vi "Mathcad 15 writeV.vi"(8 "error in (no error)":errorcluster, 10 "file text":string, 11 "DesignRequest":T1={"Project Folder"=path "", "Method Name"="", "Inputs"=[{"Label.Text"="L.Box", "Control Type"=0, "Numeric"=5.0, "Array"=[], "status"=FALSE, "Str Array"=[], "String"="", "unit"="m"}, {"Label.Text"="W.Box", "Control Type"=0, "Numeric"=2.0, "Array"=[], "status"=FALSE, "Str Array"=[], "String"="", "unit"="m"}, {"Label.Text"="H.Box", "Control Type"=0, "Numeric"=11.0, "Array"=[], "status"=FALSE, "Str Array"=[], "String"="", "unit"="m"}], "Version"=0}) -> (0 "error out":errorcluster, 2 "file text out":string)   [LabVIEW 2012, in "Design Server.lvlib"]
uses:
  Design Server.lvlib
  Design Request.ctl
  Variable cluster.ctl
panel:
  out "unit":string
  out "Array":string[](array[string])
  out "indexes":i32[](array[numeric])
  out "Regions":string[](array[string])
  # "replace existing region"
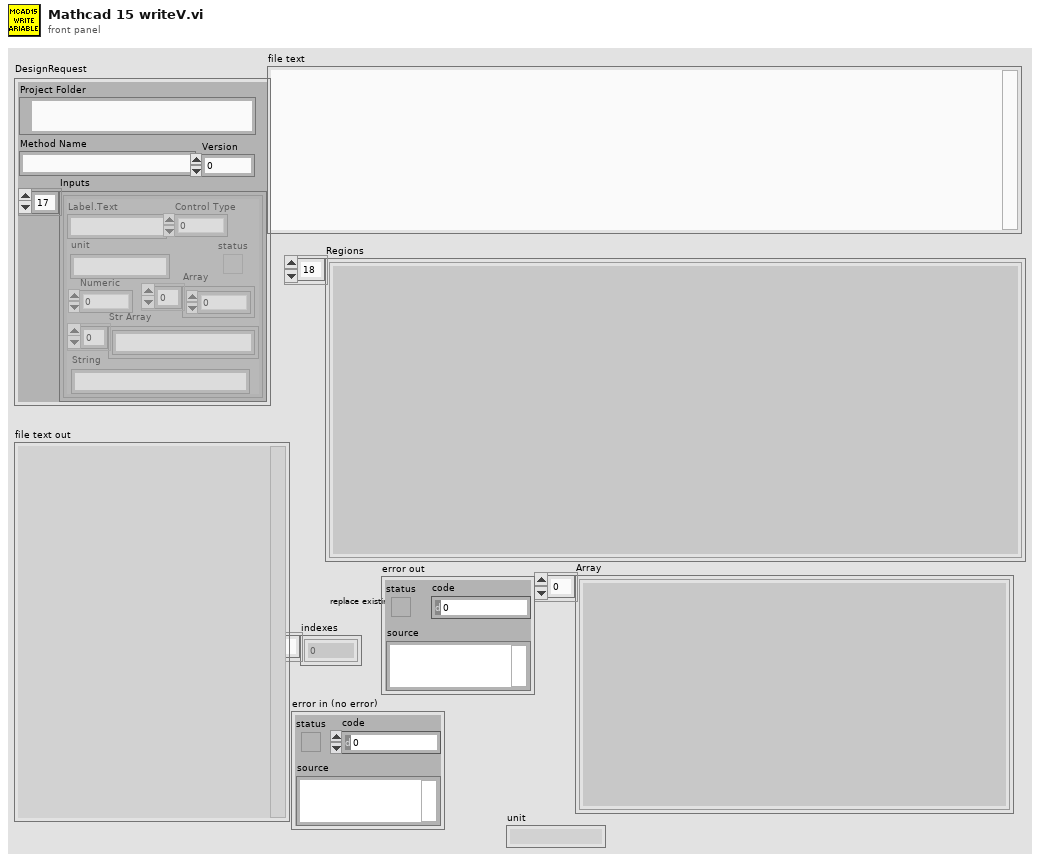
[diagram p1: front panel]
types:
  T1 = typedef "Design Server.lvlib/Design Request.ctl" = cluster{"Project Folder":path, "Method Name":string, "Inputs":T2, "Version":i32}
  T2 = typedef "Design Server.lvlib/Variable cluster.ctl" = cluster{"Label.Text":string, "Control Type":u32, "Numeric":dbl, "Array":dbl[], "status":bool, "Str Array":string[], "String":string, "unit":string}[]
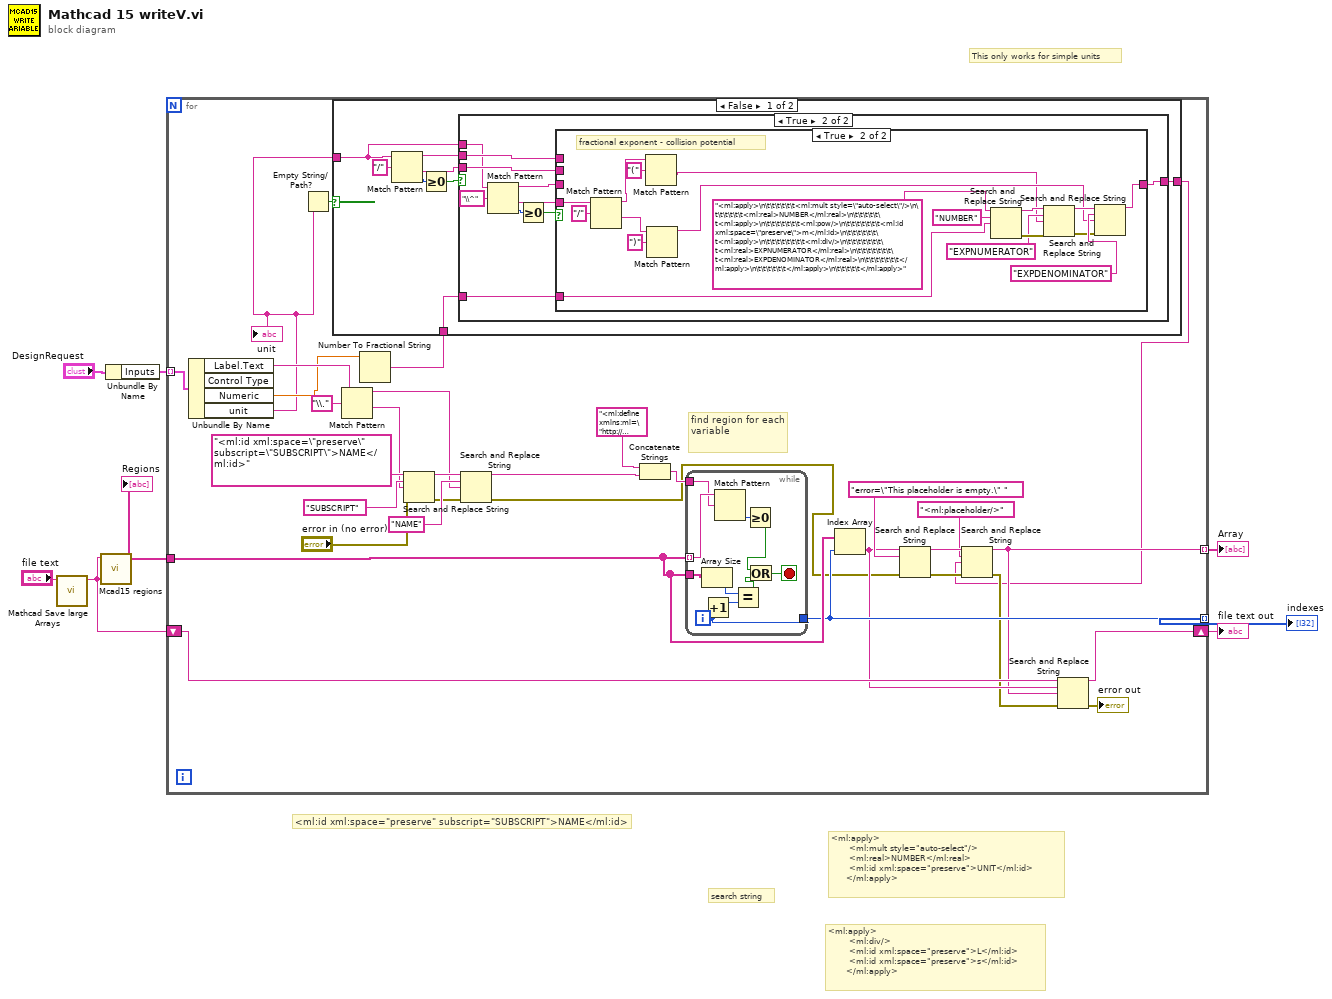
[diagram p0: block diagram]
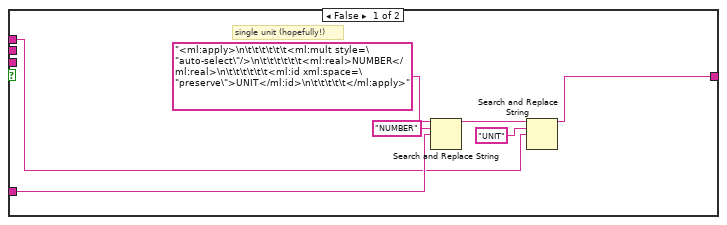
[diagram p2: hidden frame]
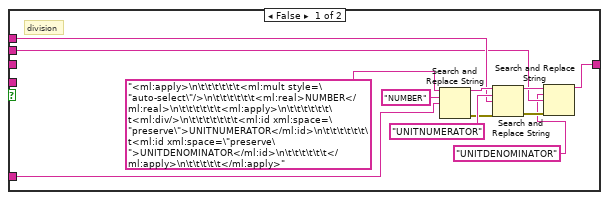
[diagram p3: hidden frame]
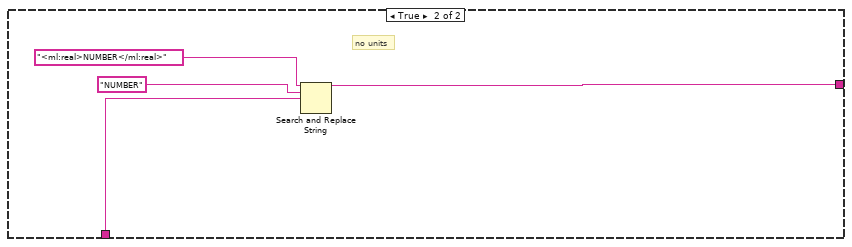
[diagram p4: hidden frame]
diagram:
  # "This only works for simple units"
  # "<ml:apply>\n\t\t\t\t\t\t\t<ml:div/>\n\t\t\t\t\t\t\t<ml:id xml:space=\"preserve\">L</ml:id>\n\t\t\t\t\t\t\t<ml:id xml:space=\"preserve\">s</ml:id>\n\t\t\t\t\t\t</ml:apply>"
  # "<ml:apply>\n\t\t\t\t\t\t<ml:mult style=\"auto-select\"/>\n\t\t\t\t\t\t<ml:real>NUMBER</ml:real>\n\t\t\t\t\t\t<ml:id xml:space=\"preserve\">UNIT</ml:id>\n\t\t\t\t\t</ml:apply>"
  # "search string"
  # "<ml:id xml:space=\"preserve\" subscript=\"SUBSCRIPT\">NAME</ml:id>"
  n1 = call "Mathcad Save large Arrays.vi"("file text"="file text") -> ("file text w save large arrays"=w1:string)  [unwired: 9 in, 1 out]
  n2 = call "Mcad15 regions.vi"("file text in"=w1) -> ("Regions"=w3:string[])  [unwired: 9 in, 1 out]
  "Regions" <- w3
  n3 = Unbundle By Name("DesignRequest") -> ("Inputs"=w7:T2)
  n4 = for {
    tunnel: w7 -> [w40] mode=indexing
    tunnel: w3 -> [w29]
    tunnel: [w28] -> w6 mode=indexing
    tunnel: [w19] -> w5 mode=indexing
    shift-right: [w21] -> w4
    shift-left: w1 -> [w22]
    # "find region for each variable"
    n5 = Unbundle By Name(w40) -> ("Label.Text"=w39:string, "Numeric"=w23:dbl, "unit"=w11:string)  [unwired: 1 out]
    "unit" <- w11
    n6 = Empty String/Path?(string/path=w11) -> (empty?=w13:bool)
    n7 = Match Pattern(string=w39, regular expression="\\.") -> (before substring=w32:string, after substring=w35:string)  [unwired: 1 in, 2 out]
    n8 = Number To Fractional String(number=w23) -> (F-format string=w12:string)  [unwired: 3 in]
    n9 = case shown="False" w13 {
      tunnel: w12 -> [w44 w98]
      tunnel: [w43 w96] -> w10
      tunnel: w11 -> [w45 _]
      frame False {
        n10 = Match Pattern(string=w45, regular expression="/") -> (before substring=w42:string, after substring=w41:string, offset past match=w47:i32)  [unwired: 1 in, 1 out]
        n11 = Greater Or Equal To 0?(x=w47) -> (x >= 0?=w46:bool)
        n12 = case shown="True" w46 {
          tunnel: w45 -> [w50 w58]
          tunnel: w44 -> [w53 w65]
          tunnel: [w49 w62] -> w43
          tunnel: w42 -> [_ w64]
          tunnel: w41 -> [_ w63]
          frame False {
            # "single unit (hopefully!)"
            n13 = Search and Replace String(input string="<ml:apply>\n\t\t\t\t\t\t<ml:mult style=\"auto-select\"/>\n\t\t\t\t\t\t<ml:real>NUMBER</ml:real>\n\t\t\t\t\t\t<ml:id xml:space=\"preserve\">UNIT</ml:id>\n\t\t\t\t\t</ml:apply>", search string="NUMBER", replace string=w53) -> (result string=w51:string)  [unwired: 5 in, 3 out]
            n14 = Search and Replace String(input string=w51, search string="UNIT", replace string=w50) -> (result string=w49:string)  [unwired: 5 in, 3 out]
          }
          frame True {
            n15 = Match Pattern(string=w58, regular expression="\\^") -> (before substring=w57:string, after substring=w56:string, offset past match=w61:i32)  [unwired: 1 in, 1 out]
            n16 = Greater Or Equal To 0?(x=w61) -> (x >= 0?=w60:bool)
            n17 = case shown="True" w60 {
              tunnel: w65 -> [w73 w87]
              tunnel: w64 -> [w72 _]
              tunnel: w63 -> [w68 _]
              tunnel: [w66 w86] -> w62
              tunnel: w57 -> [_ _]
              tunnel: w56 -> [_ w84]
              frame False {
                # "division"
                n18 = Search and Replace String(input string="<ml:apply>\n\t\t\t\t\t\t<ml:mult style=\"auto-select\"/>\n\t\t\t\t\t\t<ml:real>NUMBER</ml:real>\n\t\t\t\t\t\t<ml:apply>\n\t\t\t\t\t\t\t<ml:div/>\n\t\t\t\t\t\t\t<ml:id xml:space=\"preserve\">UNITNUMERATOR</ml:id>\n\t\t\t\t\t\t\t<ml:id xml:space=\"preserve\">UNITDENOMINATOR</ml:id>\n\t\t\t\t\t\t</ml:apply>\n\t\t\t\t\t</ml:apply>", search string="NUMBER", replace string=w73) -> (result string=w75:string, error out=w69:errorcluster)  [unwired: 5 in, 2 out]
                n19 = Search and Replace String(input string=w75, search string="UNITNUMERATOR", replace string=w72, error in=w69) -> (result string=w71:string, error out=w70:errorcluster)  [unwired: 4 in, 2 out]
                n20 = Search and Replace String(input string=w71, search string="UNITDENOMINATOR", replace string=w68, error in=w70) -> (result string=w66:string)  [unwired: 4 in, 3 out]
              }
              frame True {
                # "fractional exponent - collision potential"
                n21 = Match Pattern(string=w84, regular expression="/") -> (before substring=w78:string, after substring=w82:string)  [unwired: 1 in, 2 out]
                n22 = Match Pattern(string=w78, regular expression="(") -> (after substring=w79:string)  [unwired: 1 in, 3 out]
                n23 = Match Pattern(string=w82, regular expression=")") -> (before substring=w81:string)  [unwired: 1 in, 3 out]
                n24 = Search and Replace String(input string="<ml:apply>\n\t\t\t\t\t\t<ml:mult style=\"auto-select\"/>\n\t\t\t\t\t\t<ml:real>NUMBER</ml:real>\n\t\t\t\t\t\t<ml:apply>\n\t\t\t\t\t\t\t<ml:pow/>\n\t\t\t\t\t\t\t<ml:id xml:space=\"preserve\">m</ml:id>\n\t\t\t\t\t\t\t<ml:apply>\n\t\t\t\t\t\t\t\t<ml:div/>\n\t\t\t\t\t\t\t\t<ml:real>EXPNUMERATOR</ml:real>\n\t\t\t\t\t\t\t\t<ml:real>EXPDENOMINATOR</ml:real>\n\t\t\t\t\t\t\t</ml:apply>\n\t\t\t\t\t\t</ml:apply>\n\t\t\t\t\t</ml:apply>", search string="NUMBER", replace string=w87) -> (result string=w90:string, error out=w94:errorcluster)  [unwired: 5 in, 2 out]
                n25 = Search and Replace String(input string=w90, search string="EXPNUMERATOR", replace string=w79, error in=w94) -> (result string=w92:string, error out=w93:errorcluster)  [unwired: 4 in, 2 out]
                n26 = Search and Replace String(input string=w92, search string="EXPDENOMINATOR", replace string=w81, error in=w93) -> (result string=w86:string)  [unwired: 4 in, 3 out]
              }
            }
          }
        }
      }
      frame True {
        # "no units"
        n27 = Search and Replace String(input string="<ml:real>NUMBER</ml:real>", search string="NUMBER", replace string=w98) -> (result string=w96:string)  [unwired: 5 in, 3 out]
      }
    }
    n28 = Search and Replace String(input string="<ml:id xml:space=\"preserve\" subscript=\"SUBSCRIPT\">NAME</ml:id>", search string="SUBSCRIPT", replace string=w35, error in="error in (no error)") -> (result string=w34:string, error out=w16:errorcluster)  [unwired: 4 in, 2 out]
    n29 = Search and Replace String(input string=w34, search string="NAME", replace string=w32, error in=w16) -> (result string=w31:string, error out=w9:errorcluster)  [unwired: 4 in, 2 out]
    n30 = Concatenate Strings("<ml:define xmlns:ml=\"http://schemas.mathsoft.com/math30\">\n\t\t\t\t\t", w31) -> (w30:string)
    n31 = while {
      tunnel: w29 -> [w109] mode=indexing
      tunnel: w30 -> [w108]
      tunnel: w29 -> [w105]
      tunnel: [w100] -> w28
      i -> [w100]
      stop <- w101 stop-if-true
      n32 = Array Size(array=w105) -> (size(s)=w104:i32)
      n33 = Increment(x=w100) -> (x+1=w103:i32)
      n34 = Match Pattern(string=w109, regular expression=w108) -> (offset past match=w107:i32)  [unwired: 1 in, 3 out]
      n35 = Equal?(x=w104, y=w103) -> (x = y?=w102:bool)
      n36 = Greater Or Equal To 0?(x=w107) -> (x >= 0?=w106:bool)
      n37 = Or(x=w106, y=w102) -> (x .or. y?=w101:bool)
    }
    n38 = Index Array(array=w29, index=w28) -> (element=w20:string)
    n39 = Search and Replace String(input string=w20, search string="error=\"This placeholder is empty.\" ", error in=w9) -> (result string=w25:string, error out=w26:errorcluster)  [unwired: 5 in, 2 out]
    n40 = Search and Replace String(input string=w25, search string="<ml:placeholder/>", replace string=w10, error in=w26) -> (result string=w19:string, error out=w18:errorcluster)  [unwired: 4 in, 2 out]
    n41 = Search and Replace String(input string=w22, search string=w20, replace string=w19, error in=w18) -> (result string=w21:string, error out=→"error out":errorcluster)  [unwired: 4 in, 2 out]
  }
  "indexes" <- w6
  "Array" <- w5
  "file text out" <- w4
